vi "EF_Preprocessing.vi"(8 "Preprocessing params":T3, 10 "EOG channels":i32[](array[numeric]), 11 "EEG data in":waveform(dbl)[](array[waveform])) -> (3 "EEG data out":waveform(dbl)[](array[waveform]))   [LabVIEW 2016, in "Feature Extraction.lvlib"]
uses:
  Feature Extraction.lvlib
  EF_SpatialFilter.ctl
  EF_FrequencyFilter.ctl
panel:
  # "This VI is a part of BCI Design library, http://www.ru-bci.org \nCopyright © 2020, Sotnikov Peter, All rights reserved. License: GNU GPLv3"
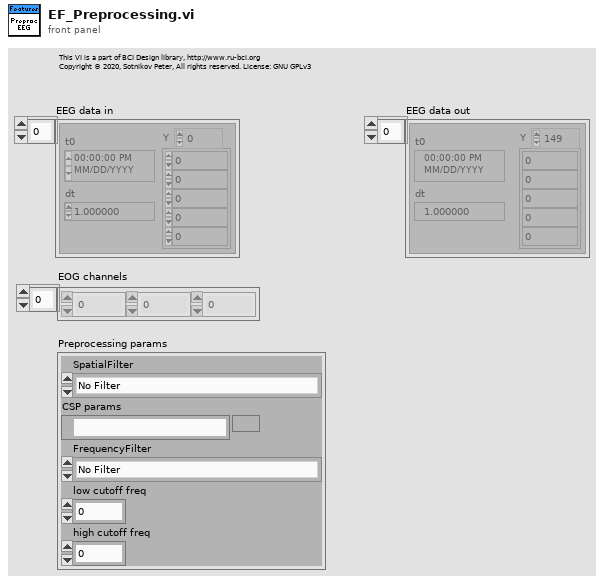
[diagram p1: front panel]
types:
  T1 = typedef "Feature Extraction.lvlib/EF_SpatialFilter.ctl" = enum16{"No Filter", "Common Average Reference", "Common Spatial Pattern Filter", "Removal of EOG Artifacts"}
  T2 = typedef "Feature Extraction.lvlib/EF_FrequencyFilter.ctl" = enum16{"No Filter", "Kaiser Filter"}
  T3 = cluster{"SpatialFilter":T1, "CSP params":path, "FrequencyFilter":T2, "low cutoff freq":dbl, "high cutoff freq":dbl}
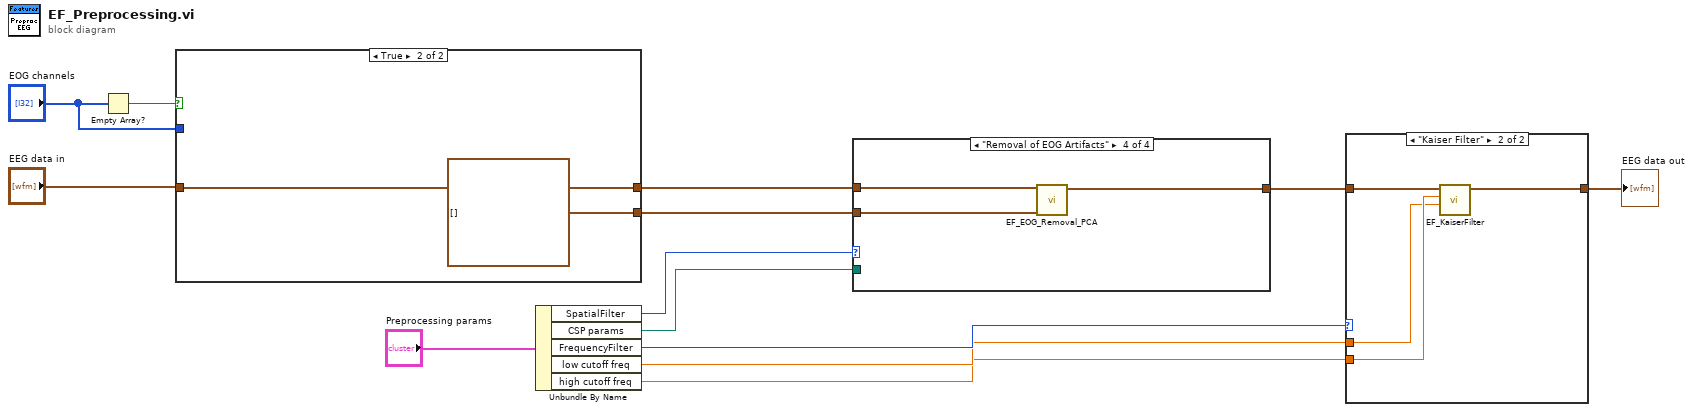
[diagram p0: block diagram]
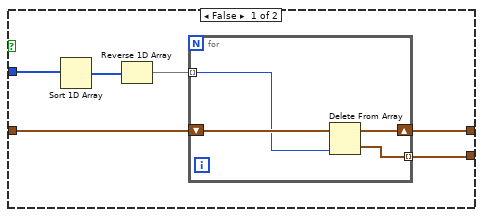
[diagram p2: hidden frame]
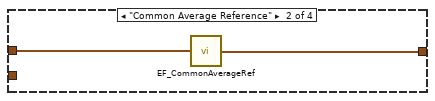
[diagram p5: hidden frame]
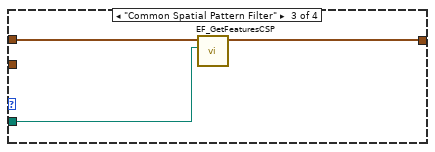
[diagram p6: hidden frame]
diagram:
  n1 = Empty Array?(array="EOG channels") -> (empty?=w5:bool)
  n2 = case shown="True" w5 {
    tunnel: "EEG data in" -> [w19 w25]
    tunnel: "EOG channels" -> [w18 _]
    tunnel: [w15 w25] -> w2
    tunnel: [w14 waveform(dbl)[] []] -> w1
    frame False {
      n3 = Sort 1D Array(array=w18) -> (sorted array=w17:i32[])
      n4 = Reverse 1D Array(array=w17) -> (reversed array=w16:i32[])
      n5 = for {
        tunnel: w16 -> [w20] mode=indexing
        shift-right: [w22] -> w15
        shift-left: w19 -> [w23]
        tunnel: [w21] -> w14 mode=indexing
        n6 = Delete From Array(array=w23, index=w20) -> (deleted portion=w21:waveform(dbl), array with subset deleted=w22:waveform(dbl)[])  [unwired: 1 in]
      }
    }
    frame True {
    }
  }
  n7 = Unbundle By Name("Preprocessing params") -> ("SpatialFilter"=w12:T1, "CSP params"=w11:path, "FrequencyFilter"=w10:T2, "low cutoff freq"=w8:dbl, "high cutoff freq"=w7:dbl)
  n8 = case shown="\"Removal of EOG Artifacts\"" w12 {
    tunnel: [w26 w28 w30 w34] -> w9
    tunnel: w11 -> [_ _ w31 _]
    tunnel: w2 -> [w26 w27 w29 w33]
    tunnel: w1 -> [_ _ _ w32]
    frame "No Filter", Default {
    }
    frame "Common Average Reference" {
      n9 = call "EF_CommonAverageRef.vi"("Array Of Waveforms in"=w27) -> ("Array Waveforms out"=w28:waveform(dbl)[])
    }
    frame "Common Spatial Pattern Filter" {
      n10 = call "EF_GetFeaturesCSP.vi"("CSP filter file"=w31, "Array Of Waveforms in"=w29) -> ("Array Of Waveforms out"=w30:waveform(dbl)[])  [unwired: 8 in, 1 out]
    }
    frame "Removal of EOG Artifacts" {
      n11 = call "EF_EOG_Removal_PCA.vi"("EOG"=w32, "EEG"=w33) -> ("EEG out"=w34:waveform(dbl)[])  [unwired: 9 in]
    }
  }
  n12 = case shown="\"Kaiser Filter\"" w10 {
    tunnel: w9 -> [w35 w39]
    tunnel: w8 -> [_ w37]
    tunnel: w7 -> [_ w38]
    tunnel: [w35 w36] -> w6
    frame "No Filter", Default {
    }
    frame "Kaiser Filter" {
      n13 = call "EF_KaiserFilter.vi"("low cutoff freq: fl"=w37, "high cutoff freq: fh"=w38, "Array Of Waveforms in"=w39) -> ("Filtered Waveforms"=w36:waveform(dbl)[])  [unwired: 7 in, 1 out]
    }
  }
  "EEG data out" <- w6
